vi "Set Injected Value static.vi"(8 "error in (no error)":errorcluster, 10 "Value":T1, 11 "Fault-Injection_DBL in":refnum<class "Fault-Injection_DBL.lvclass">) -> (0 "error out":errorcluster, 3 "Fault-Injection_DBL out":refnum<class "Fault-Injection_DBL.lvclass">)   [LabVIEW 2021, in "Fault-Injection_DBL.lvclass"]
uses:
  Fault-Injection_DBL.lvclass
  Value Type.ctl
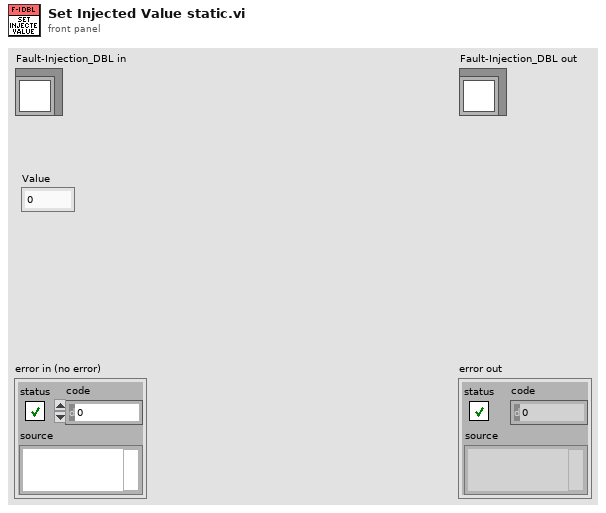
[diagram p1: front panel]
types:
  T1 = typedef "Fault-Injection_DBL.lvclass/Value Type.ctl" = dbl
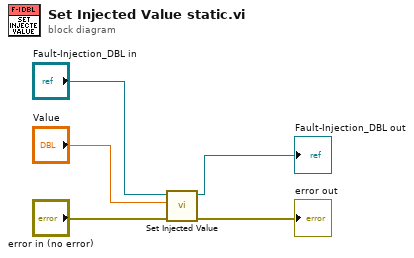
[diagram p0: block diagram]
diagram:
  n1 = call-dynamic "Set Injected Value.vi"("error in (no error)"="error in (no error)", "Value"="Value", "Fault-Injection_Boolean in"="Fault-Injection_DBL in") -> ("error out"=→"error out":errorcluster, "Fault-Injection_Boolean out"=→"Fault-Injection_DBL out":refnum<class "Fault-Injection_DBL.lvclass">)  [unwired: 7 in]
